vi "SW_Convert_data_from_old_format_save.vi"(7 "Time Stamp in":timestamp format="%<%.0X\n%x>T", 8 "error in (no error)":errorcluster, 9 "File name":string="Loaded file of previous version", 10 "Researcher name":string="Researcher", 11 "Loaded data in":T2) -> (0 "error out":errorcluster, 3 "Loaded data out":T1)   [LabVIEW 2018, in "Tracker.lvlib"]
uses:
  Tracker.lvlib
  Controls/CTL_Loaded_data_output_(offline).ctl
  Controls/CTL_Settings_cluster.ctl
  Controls/CTL_Histogram_parameters.ctl
  Controls/CTL_Filter_selector.ctl
  Controls/CTL_Acquisition_speed_selector.ctl
  Controls/CTL_Segmented_plot_parameters.ctl
  Controls/CTL_IO_params_cluster.ctl
  Controls/CTL_Conditions_Array.ctl
  Controls/CTL_Conditions_Cluster.ctl
  Controls/CTL_Condition_type.ctl
  Controls/CTL_Comparison_type.ctl
  Controls/CTL_Validity_check_criteria.ctl
  Controls/CTL_Response_info.ctl
  Controls/CTL_Condition_response_type.ctl
  Controls/CTL_Reponse_port_info.ctl
  Controls/CTL_Calibration_parameters.ctl
  Controls/CTL_Dispenser_calibration_info.ctl
  <vilib>/Analysis/baseanly.llb/Mean (DBL).vi
  <vilib>/Analysis/NI_AALBase.lvlib
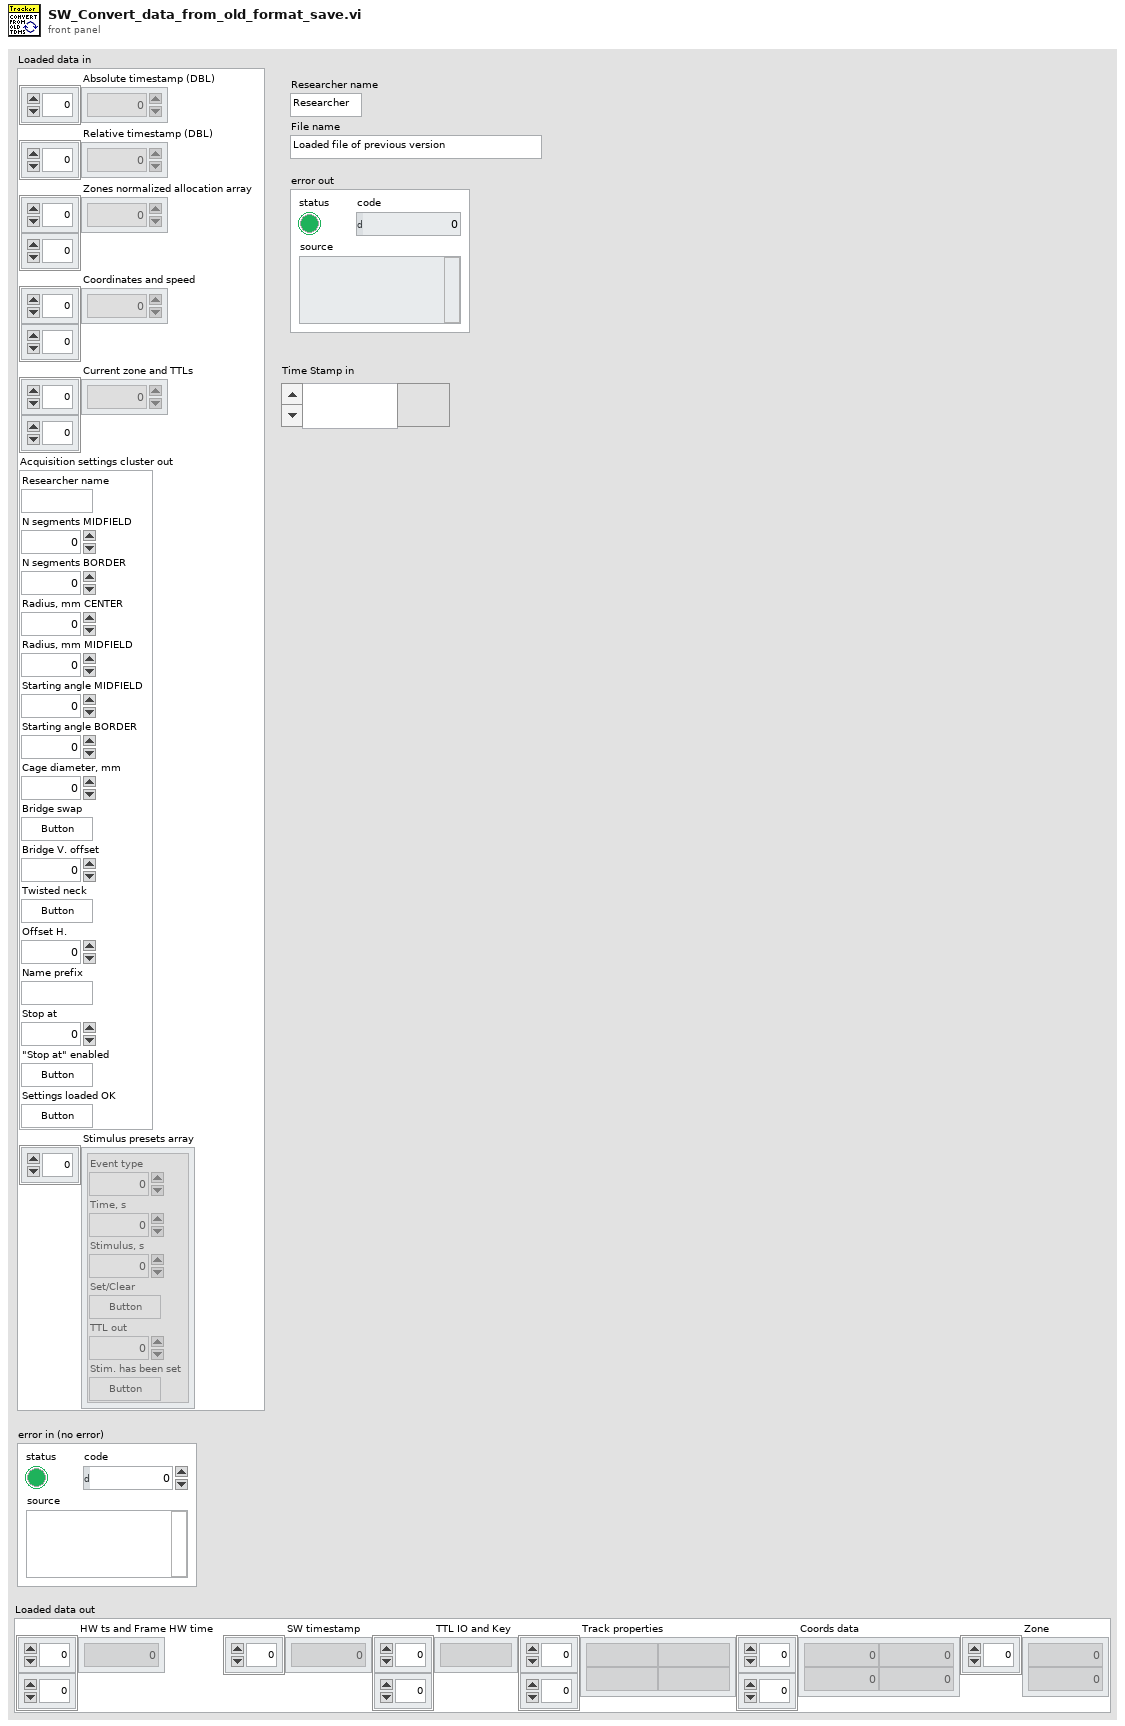
[diagram p1: front panel]
types:
  T1 = typedef "Tracker.lvlib/CTL_Loaded_data_output_(offline).ctl" = cluster{"HW ts and Frame HW time":u32[][], "SW timestamp":dbl[], "TTL IO and Key":string[][], "Track properties":string[][], "Coords data":dbl[][], "Zone":i8[]}
  T2 = cluster{"Absolute timestamp (DBL)":dbl[], "Relative timestamp (DBL)":dbl[], "Zones normalized allocation array":dbl[][], "Coordinates and speed":dbl[][], "Current zone and TTLs":u8[][], "Acquisition settings cluster out":cluster{"Researcher name":string, "N segments MIDFIELD":u8, "N segments BORDER":u8, "Radius, mm CENTER":u16, "Radius, mm MIDFIELD":u16, "Starting angle MIDFIELD":i16, "Starting angle BORDER":i16, "Cage diameter, mm":u16, "Bridge swap":bool, "Bridge V. offset":sgl, "Twisted neck":bool, "Offset H.":sgl, "Name prefix":string, "Stop at":dbl, "\"Stop at\" enabled":bool, "Settings loaded OK":bool}, "Stimulus presets array":cluster{"Event type":u16, "Time, s":sgl, "Stimulus, s":sgl, "Set/Clear":bool, "TTL out":u16, "Stim. has been set":bool}[]}
  T3 = typedef "Tracker.lvlib/CTL_Segmented_plot_parameters.ctl" = cluster{"Cage diameter, mm":u16, "Starting angle MIDFIELD":i16, "Starting angle BORDER":i16, "Radius, mm CENTER":u16, "Radius, mm MIDFIELD":u16, "N segments MIDFIELD":u8, "N segments BORDER":u8, "R-gap, mm":sgl, "Bridge swap":bool, "Bridge H. offset":sgl, "Bridge V. offset":sgl, "Twisted neck":bool, "Alt. magn. orientation":bool, "Sensor board size":enum16{"Small", "Large"}}
  T4 = typedef "Tracker.lvlib/CTL_Settings_cluster.ctl" = cluster{"Defaults":cluster{"Default User":dbl, "VISA Resource Name ":string, "Histogram parameters":T5}, "Recording and saving":cluster{"Researcher name":string, "Name prefix":string, "Data post-processing":T6, "Stop at":dbl, "\"Stop at\" enabled":bool, "Default save folder path":path, "Acquisition FPS":T7}, "Geometry":T3, "IO parameters":T8, "Conditions presets array":T9, "Calibration parameters":T17, "Settings loaded OK":bool}
  T5 = typedef "Tracker.lvlib/CTL_Histogram_parameters.ctl" = cluster{"max":dbl, "min":dbl, "# bins":i32, "threshold":dbl, "thr. type":enum16{"higher accepted", "lower accepted"}}
  T6 = typedef "Tracker.lvlib/CTL_Filter_selector.ctl" = cluster{"Filter type":enum16{"None", "Savitzky-Golay"}, "Length":i32, "Order":i32}
  T7 = typedef "Tracker.lvlib/CTL_Acquisition_speed_selector.ctl" = enum16{"Max", "Optimal", "Eco"}
  T8 = typedef "Tracker.lvlib/CTL_IO_params_cluster.ctl" = cluster{"IO general config.":u16, "IO 1 configuration":u16, "IO 2 configuration":u16, "IO 3 configuration":u16, "IO 4 configuration":u16, "Activate ext. RS-232":u16, "IO inversion config.":u16, "Sync capability":u8}
  T9 = typedef "Tracker.lvlib/CTL_Conditions_Array.ctl" = T10[]
  T10 = typedef "Tracker.lvlib/CTL_Conditions_Cluster.ctl" = cluster{"Enabled":bool, "Name":string, "Specifier(s)":cluster{"Specifier enabled":bool, "Condition type":T11, "Comparison type":T12, "Value":dbl, "Validity criteria(s)":cluster{"V. check enabled":bool, "Criteria":T13, "Validity value":dbl}[]}[], "Response":T14, "Has been set":bool}
  T11 = typedef "Tracker.lvlib/CTL_Condition_type.ctl" = enum16{"Speed", "Zone", "Angle to wall"}
  T12 = typedef "Tracker.lvlib/CTL_Comparison_type.ctl" = enum16{"Less", "Less or Equal", "Equal", "Greater or Equal", "Greater", "Not Equal"}
  T13 = typedef "Tracker.lvlib/CTL_Validity_check_criteria.ctl" = enum16{"Running bout (seconds)", "Running bout (meters)"}
  T14 = typedef "Tracker.lvlib/CTL_Response_info.ctl" = cluster{"Response type":T15, "TTL port":T16, "TTL pulse length, ms":dbl}
  T15 = typedef "Tracker.lvlib/CTL_Condition_response_type.ctl" = enum16{"None", "Air puff", "Liquid reward"}
  T16 = typedef "Tracker.lvlib/CTL_Reponse_port_info.ctl" = enum16{"Port 1", "Port 2", "Port 3", "Port 4"}
  T17 = typedef "Tracker.lvlib/CTL_Calibration_parameters.ctl" = cluster{"Timing calibration sw/hw":dbl, "True FPS":dbl, "True frame time, s":dbl, "Disp. calibration info":T18}
  T18 = typedef "Tracker.lvlib/CTL_Dispenser_calibration_info.ctl" = cluster{"Channel":u8, "Speed, µl per ms":dbl}[]
  T19 = cluster{"Researcher name":string, "N segments MIDFIELD":u8, "N segments BORDER":u8, "Radius, mm CENTER":u16, "Radius, mm MIDFIELD":u16, "Starting angle MIDFIELD":i16, "Starting angle BORDER":i16, "Cage diameter, mm":u16, "Bridge swap":bool, "Bridge V. offset":sgl, "Twisted neck":bool, "Offset H.":sgl, "Name prefix":string, "Stop at":dbl, "\"Stop at\" enabled":bool, "Settings loaded OK":bool}
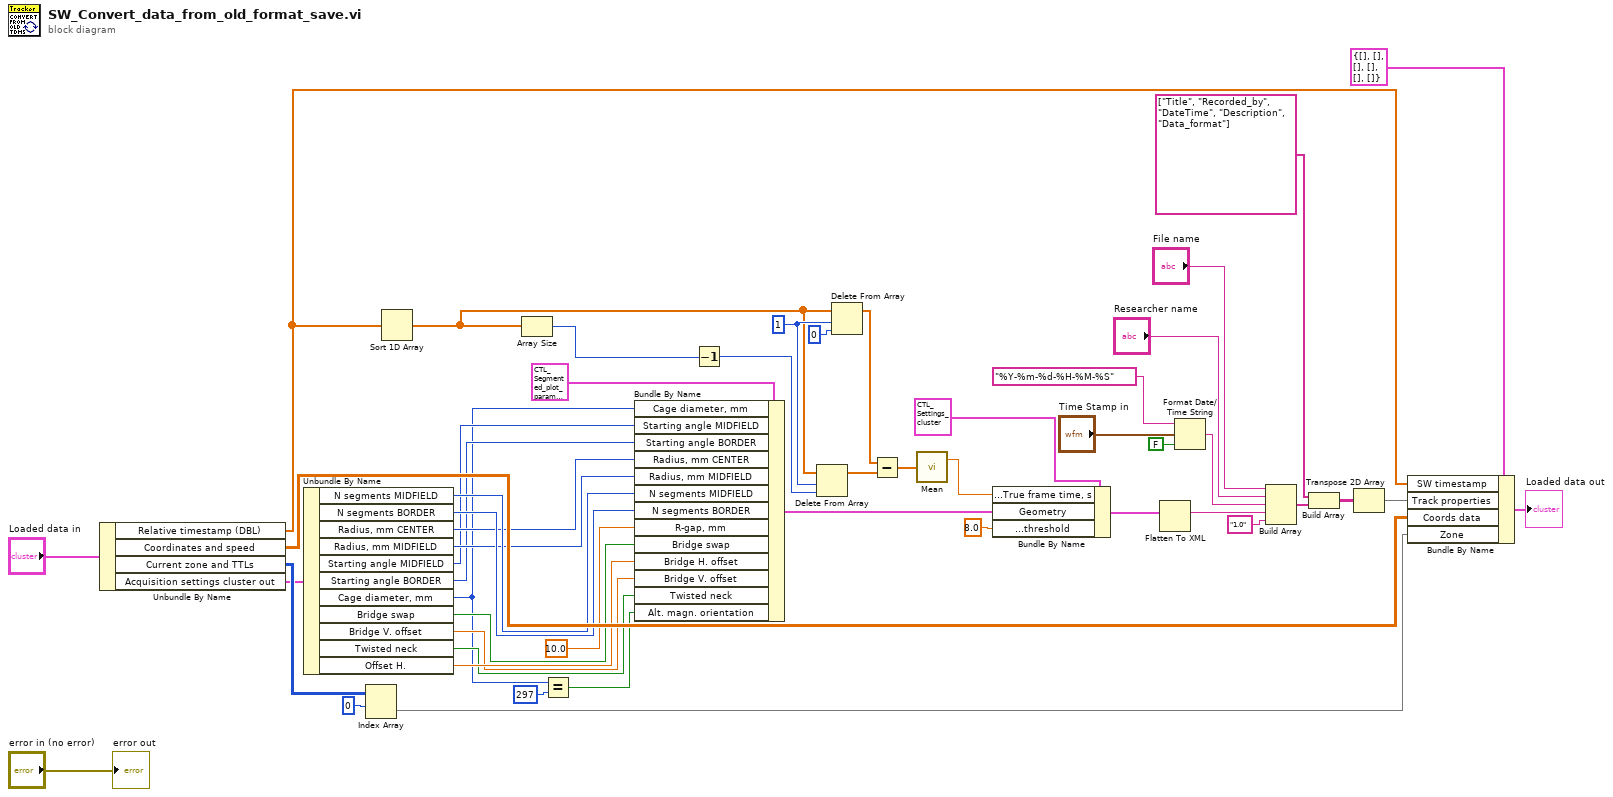
[diagram p0: block diagram]
diagram:
  w23 = 1 ("length")
  n1 = Unbundle By Name("Loaded data in") -> ("Relative timestamp (DBL)"=w18:dbl[], "Coordinates and speed"=w47:dbl[][], "Current zone and TTLs"=w46:u8[][], "Acquisition settings cluster out"=w40:T19)
  n2 = Unbundle By Name(w40) -> ("N segments MIDFIELD"=w39:u8, "N segments BORDER"=w38:u8, "Radius, mm CENTER"=w37:u16, "Radius, mm MIDFIELD"=w36:u16, "Starting angle MIDFIELD"=w35:i16, "Starting angle BORDER"=w34:i16, "Cage diameter, mm"=w29:u16, "Bridge swap"=w33:bool, "Bridge V. offset"=w30:sgl, "Twisted neck"=w31:bool, "Offset H."=w32:sgl)
  n3 = Index Array(array=w46, index (row)=0) -> (element=w44:u8[])  [unwired: 1 in]
  n4 = Sort 1D Array(array=w18) -> (sorted array=w17:dbl[])
  n5 = Array Size(array=w17) -> (size(s)=w24:i32)
  n6 = Equal?(x=w29, y=u16 297) -> (x = y?=w27:bool)
  n7 = Bundle By Name(cluster=T3 {"Cage diameter, mm"=180, "Starting angle MIDFIELD"=0, "Starting angle BORDER"=0, "Radius, mm CENTER"=30, "Radius, mm MIDFIELD"=75, "N segments MIDFIELD"=2, "N segments BORDER"=4, "R-gap, mm"=0.0, "Bridge swap"=FALSE, "Bridge H. offset"=0.0, "Bridge V. offset"=0.0, "Twisted neck"=FALSE, "Alt. magn. orientation"=FALSE, "Sensor board size"=enum."Small"} ("Geometry"), "Cage diameter, mm"=w29, "Starting angle MIDFIELD"=w35, "Starting angle BORDER"=w34, "Radius, mm CENTER"=w37, "Radius, mm MIDFIELD"=w36, "N segments MIDFIELD"=w39, "N segments BORDER"=w38, "R-gap, mm"=sgl 10.0, "Bridge swap"=w33, "Bridge H. offset"=w32, "Bridge V. offset"=w30, "Twisted neck"=w31, "Alt. magn. orientation"=w27) -> (w41:T3)
  n8 = Decrement(x=w24) -> (x-1=w22:i32)
  n9 = Delete From Array(array=w17, length=w23, index=w22) -> (array with subset deleted=w20:dbl[])  [unwired: 1 out]
  n10 = Delete From Array(array=w17, length=w23, index=0) -> (array with subset deleted=w21:dbl[])  [unwired: 1 out]
  n11 = Subtract(x=w21, y=w20) -> (x-y=w19:dbl[])
  n12 = call-poly <vilib>:"Mean.vi"("X"=w19) -> ("mean"=w16:dbl)  [unwired: 1 out]
  n13 = Bundle By Name(cluster=T4 {"Defaults"={"Default User"=0.0, "VISA Resource Name "="Tracker", "Histogram parameters"={"max"=300.0, "min"=0.0, "# bins"=10, "threshold"=8.0, "thr. type"=enum."higher accepted"}}, "Recording and saving"={"Researcher name"="Researcher", "Name prefix"="Track", "Data post-processing"={"Filter type"=enum."Savitzky-Golay", "Length"=31, "Order"=3}, "Stop at"=0.0, "\"Stop at\" enabled"=FALSE, "Default save folder path"=path "", "Acquisition FPS"=enum."Max"}, "Geometry"={"Cage diameter, mm"=180, "Starting angle MIDFIELD"=0, "Starting angle BORDER"=0, "Radius, mm CENTER"=30, "Radius, mm MIDFIELD"=75, "N segments MIDFIELD"=2, "N segments BORDER"=4, "R-gap, mm"=0.0, "Bridge swap"=FALSE, "Bridge H. offset"=0.0, "Bridge V. offset"=0.0, "Twisted neck"=FALSE, "Alt. magn. orientation"=FALSE, "Sensor board size"=enum."Small"}, "IO parameters"={"IO general config."=12, "IO 1 configuration"=1, "IO 2 configuration"=1, "IO 3 configuration"=0, "IO 4 configuration"=0, "Activate ext. RS-232"=0, "IO inversion config."=0, "Sync capability"=1}, "Conditions presets array"=[{"Enabled"=FALSE, "Name"="", "Specifier(s)"=[], "Response"={"Response type"=enum."Air puff", "TTL port"=enum."Port 1", "TTL pulse length, ms"=0.0}, "Has been set"=FALSE}, {"Enabled"=FALSE, "Name"="", "Specifier(s)"=[], "Response"={"Response type"=enum."Air puff", "TTL port"=enum."Port 1", "TTL pulse length, ms"=0.0}, "Has been set"=FALSE}, {"Enabled"=FALSE, "Name"="", "Specifier(s)"=[], "Response"={"Response type"=enum."Air puff", "TTL port"=enum."Port 1", "TTL pulse length, ms"=0.0}, "Has been set"=FALSE}, {"Enabled"=FALSE, "Name"="", "Specifier(s)"=[], "Response"={"Response type"=enum."Air puff", "TTL port"=enum."Port 1", "TTL pulse length, ms"=0.0}, "Has been set"=FALSE}, {"Enabled"=FALSE, "Name"="", "Specifier(s)"=[], "Response"={"Response type"=enum."Air puff", "TTL port"=enum."Port 1", "TTL pulse length, ms"=0.0}, "Has been set"=FALSE}, {"Enabled"=FALSE, "Name"="", "Specifier(s)"=[], "Response"={"Response type"=enum."Air puff", "TTL port"=enum."Port 1", "TTL pulse length, ms"=0.0}, "Has been set"=FALSE}, {"Enabled"=FALSE, "Name"="", "Specifier(s)"=[], "Response"={"Response type"=enum."Air puff", "TTL port"=enum."Port 1", "TTL pulse length, ms"=0.0}, "Has been set"=FALSE}, {"Enabled"=FALSE, "Name"="", "Specifier(s)"=[], "Response"={"Response type"=enum."Air puff", "TTL port"=enum."Port 1", "TTL pulse length, ms"=0.0}, "Has been set"=FALSE}, {"Enabled"=FALSE, "Name"="", "Specifier(s)"=[], "Response"={"Response type"=enum."Air puff", "TTL port"=enum."Port 1", "TTL pulse length, ms"=0.0}, "Has been set"=FALSE}, {"Enabled"=FALSE, "Name"="", "Specifier(s)"=[], "Response"={"Response type"=enum."Air puff", "TTL port"=enum."Port 1", "TTL pulse length, ms"=0.0}, "Has been set"=FALSE}, {"Enabled"=FALSE, "Name"="", "Specifier(s)"=[], "Response"={"Response type"=enum."Air puff", "TTL port"=enum."Port 1", "TTL pulse length, ms"=0.0}, "Has been set"=FALSE}, {"Enabled"=FALSE, "Name"="", "Specifier(s)"=[], "Response"={"Response type"=enum."Air puff", "TTL port"=enum."Port 1", "TTL pulse length, ms"=0.0}, "Has been set"=FALSE}, {"Enabled"=FALSE, "Name"="", "Specifier(s)"=[], "Response"={"Response type"=enum."Air puff", "TTL port"=enum."Port 1", "TTL pulse length, ms"=0.0}, "Has been set"=FALSE}, {"Enabled"=FALSE, "Name"="", "Specifier(s)"=[], "Response"={"Response type"=enum."Air puff", "TTL port"=enum."Port 1", "TTL pulse length, ms"=0.0}, "Has been set"=FALSE}], "Calibration parameters"={"Timing calibration sw/hw"=1.0, "True FPS"=80.0, "True frame time, s"=0.0125, "Disp. calibration info"=[]}, "Settings loaded OK"=FALSE} ("Settings cluster"), "Calibration parameters.True frame time, s"=w16, "Geometry"=w41, "Defaults.Histogram parameters.threshold"=8.0) -> (w15:T4)
  n14 = Flatten To XML(anything=w15) -> (xml string=w12:string)
  n15 = Format Date/Time String(time format string (%c)="%Y-%m-%d-%H-%M-%S", seconds (now)="Time Stamp in", UTC format=FALSE) -> (date/time string=w7:string)
  n16 = Build Array("File name", "Researcher name", w7, w12, "1.0" ("element")) -> (w6:string[])
  n17 = Build Array(string[] ["Title", "Recorded_by", "DateTime", "Description", "Data_format"] ("property names"), w6) -> (w5:string[][])
  n18 = Transpose 2D Array(2D array=w5) -> (transposed array=w1:string[][])
  n19 = Bundle By Name(cluster=T1 {"HW ts and Frame HW time"=[], "SW timestamp"=[], "TTL IO and Key"=[], "Track properties"=[], "Coords data"=[], "Zone"=[]} ("Loaded data output"), "SW timestamp"=w18, "Track properties"=w1, "Coords data"=w47, "Zone"=w44) -> (→"Loaded data out":T1)
  "error out" <- "error in (no error)"
